vi "rebuild all.vi"(8 "error in (no error)":errorcluster, 10 "release (T) /debug (F)":bool, 11 "project path":path) -> (0 "error":errorcluster)   [LabVIEW 2014, in "CD model script.lvlib"]
uses:
  CD model script.lvlib
  <vilib>/AppBuilder/AB_API_Simple/Build (path).vi
  <vilib>/AppBuilder/AB_API_Simple/NI_App_Builder_API.lvlib
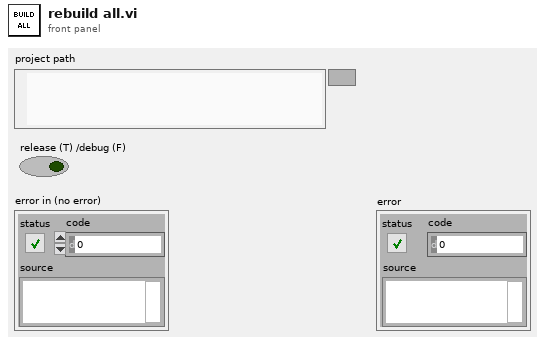
[diagram p1: front panel]
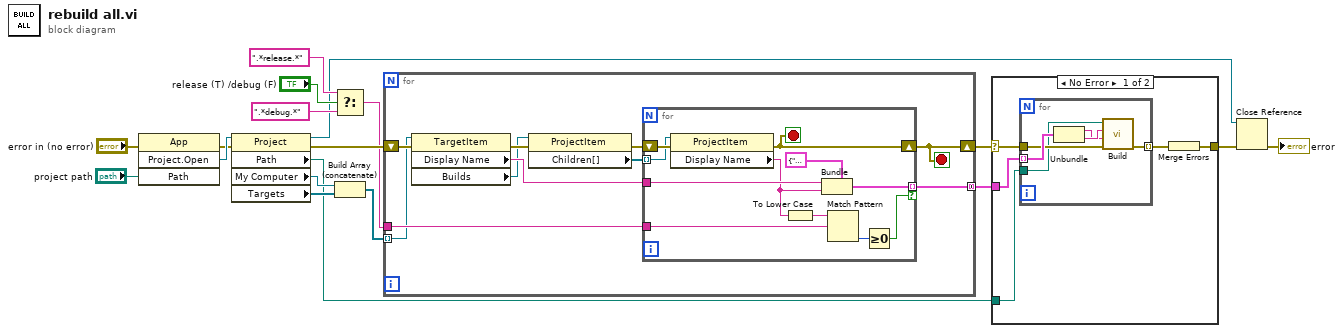
[diagram p0: block diagram]
diagram:
  n1 = invoke class="App" method="Project.Open"(error in="error in (no error)", "Path"="project path") -> (error out=w5:errorcluster, "Project:Open"=w6:refnum<vi>)  [unwired: 2 in, 2 out]
  n2 = property class="Project"(reference=w6, error in=w5) -> (reference out=w2:refnum<vi>, error out=w18:errorcluster, "Path"=w9:path, "My Computer"=w17:refnum<vi>, "Targets"=w11:refnum<vi>[])
  n3 = Select(t=".*release.*" ("regular expression"), s="release (T) /debug (F)", f=".*debug.*" ("regular expression")) -> (s? t:f=w13:string)
  n4 = Build Array (concatenate)(w17, w11) -> (w12:refnum<vi>[])
  n5 = for {
    tunnel: w13 -> [w25]
    tunnel: w12 -> [w24] mode=indexing
    shift-right: [w19] -> w8
    shift-left: w18 -> [w28]
    tunnel: [w23] -> w10 mode=concatenating
    stop <- w19 stop-if-true
    n6 = property class="TargetItem"(reference=w24, error in=w28) -> (error out=w27:errorcluster, "Display Name"=w26:string, "Builds"=w21:refnum<vi>)  [unwired: 1 out]
    n7 = property class="ProjectItem"(reference=w21, error in=w27) -> (error out=w22:errorcluster, "Children[]"=w20:refnum<vi>[])  [unwired: 1 out]
    n8 = for {
      shift-right: [w29] -> w19
      shift-left: w22 -> [w39]
      tunnel: w26 -> [w38]
      tunnel: [w36] -> w23 mode=indexing if=w34
      tunnel: w25 -> [w32]
      tunnel: w20 -> [w30] mode=indexing
      stop <- w29 stop-if-true
      n9 = property class="ProjectItem"(reference=w30, error in=w39) -> (error out=w29:errorcluster, "Display Name"=w37:string)  [unwired: 1 out]
      n10 = To Lower Case(string=w37) -> (all lower case string=w33:string)
      n11 = Bundle(cluster=cluster{"targ":string, "spec":string} {"targ"="", "spec"=""}, "targ"=w38, "spec"=w37) -> (w36:cluster{"targ":string, "spec":string})
      n12 = Match Pattern(string=w33, regular expression=w32) -> (offset past match=w35:i32)  [unwired: 1 in, 3 out]
      n13 = Greater Or Equal To 0?(x=w35) -> (x >= 0?=w34:bool)
    }
  }
  n14 = case shown="No Error" w8 {
    selector: w8 -> [w42 w51]
    tunnel: w10 -> [w44 _]
    tunnel: w9 -> [w43 _]
    tunnel: [w40 w51] -> w7
    frame No Error {
      n15 = for {
        tunnel: w44 -> [w50] mode=indexing
        tunnel: w43 -> [w48]
        tunnel: w42 -> [w49]
        tunnel: [w45] -> w41 mode=indexing
        n16 = Unbundle(w50) -> ("targ"=w46:string, "spec"=w47:string)
        n17 = call-poly <vilib>:"Build.vi"("error in (no error)"=w49, "Name of target (My Computer)"=w46, "Name of build specification (if empty: build all)"=w47, "Path to project"=w48) -> ("error out"=w45:errorcluster)  [unwired: 6 in, 1 out]
      }
      n18 = Merge Errors(w41) -> (w40:errorcluster)
    }
    frame Error {
    }
  }
  n19 = Close Reference(reference=w2, error in (no error)=w7) -> (error out=→"error":errorcluster)
